vi "Deserialise content.vi"(8 "error in (no error)":errorcluster, 10 "JSON String to decode":string, 11 "object in":refnum<class "status Message.lvclass">) -> (0 "error out":errorcluster, 3 "object out":refnum<class "status Message.lvclass">)   [LabVIEW 2018, in "ClientMessaging.lvlib" / "status Message.lvclass"]
doc: "Convert content dictionary to class private data"
uses:
  status Message.lvclass
  Status Content.ctl
  status Message.lvclass/status Message.ctl
  d97df936-6e37-42c9-9110-93c10ee1b470.vi
  d97df936-6e37-42c9-9110-93c10ee1b470.vi/d007a89c-5480-4e2f-bb8e-4b771dae55fc.vi
  d97df936-6e37-42c9-9110-93c10ee1b470.vi/0db0be89-6376-4dbe-bafb-9f4f73d06a86.vi
  <userlib>/_OpenG.lib/lvdata/lvdata.llb/Get Cluster Element by Name__ogtk.vi
  Base Classes/Message Class/Message Class.lvclass
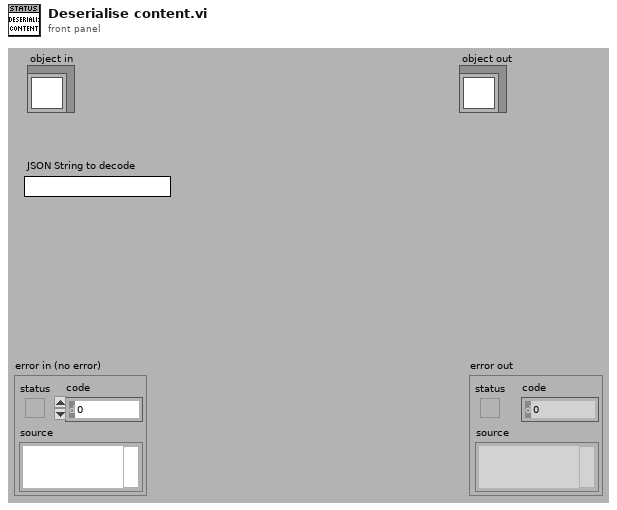
[diagram p1: front panel]
types:
  T1 = typedef "ClientMessaging.lvlib/status Message.lvclass/Status Content.ctl" = enum16{"idle", "busy", "starting"}
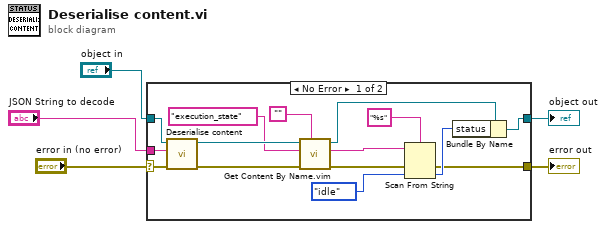
[diagram p0: block diagram]
diagram:
  n1 = case shown="No Error" "error in (no error)" {
    selector: "error in (no error)" -> [w12 w22]
    tunnel: [w6 w22] -> w4
    tunnel: [w19 w21] -> w2
    tunnel: "object in" -> [w20 w21]
    tunnel: "JSON String to decode" -> [w17 _]
    frame No Error {
      n2 = call-parent "Deserialise content.vi"("error in (no error)"=w12, "JSON String to decode"=w17, "object in"=w20) -> ("error out"=w13:errorcluster, "object out"=w18:refnum<class "status Message.lvclass">)  [unwired: 7 in]
      n3 = call "Get Content By Name.vim"("Type of content"="", "error in (no error)"=w13, "Name of Content Item"="execution_state", "Message In"=w18) -> ("error out"=w7:errorcluster, "Data Out"=w11:string, "Message Out"=w16:refnum<class "status Message.lvclass">)  [unwired: 5 in]
      n4 = Scan From String(format string="%s", input string=w11, error in=w7, default 1=Status_Content."idle" ("content")) -> (error out=w6:errorcluster, output 1=w8:T1)  [unwired: 1 in, 2 out]
      n5 = Bundle By Name(cluster=w16, "status"=w8) -> (w19:refnum<class "status Message.lvclass">)
    }
    frame Error {
    }
  }
  "error out" <- w4
  "object out" <- w2
